vi "Initialize Data.vi"(8 "error in (no error)":errorcluster, 9 "data version":T1, 10 "data":string, 11 "Core Threads Configuration in":refnum<class "Core Threads Configuration.lvclass">) -> (0 "error out":errorcluster, 3 "Core Threads Configuration out":refnum<class "Core Threads Configuration.lvclass">)   [LabVIEW 2017, in "DSF Core.lvlib" / "Core Threads Configuration.lvclass"]
uses:
  Core Threads Configuration.lvclass
  Typedefs/DSF Version Info.ctl
  Core Threads Configuration.lvclass/Core Threads Configuration.ctl
  DSF Core.lvlib
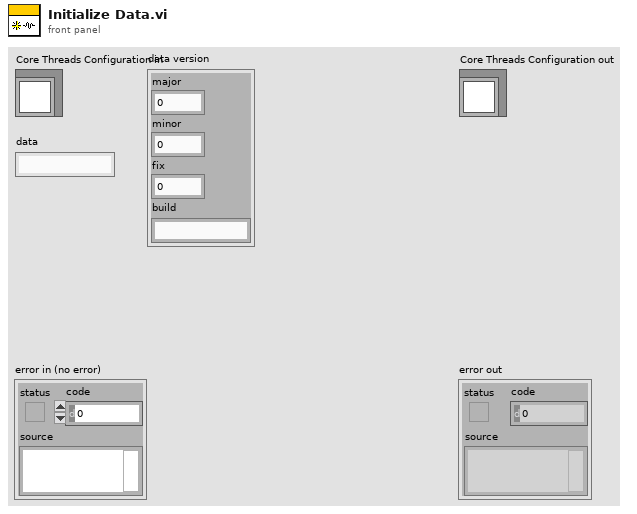
[diagram p1: front panel]
types:
  T1 = typedef "DSF Core.lvlib/DSF Version Info.ctl" = cluster{"major":i32, "minor":i32, "fix":i32, "build":string}
  T2 = cluster{"processor":i32, "priority offset":i16}[]
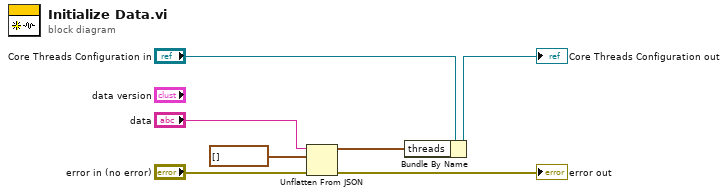
[diagram p0: block diagram]
diagram:
  n1 = Unflatten From JSON(JSON string="data", type and defaults=T2 [] ("thread configuration"), error in (no error)="error in (no error)") -> (value=w2:T2, error out=→"error out":errorcluster)  [unwired: 4 in]
  n2 = Bundle By Name(cluster="Core Threads Configuration in", "threads"=w2) -> (→"Core Threads Configuration out":refnum<class "Core Threads Configuration.lvclass">)
